vi "Select_events.vi"(8 "error in (no error)":errorcluster, 9 "Select errored events":bool, 10 "Small?":bool, 11 "Constraints":T1 {"Estimate Quality" scale=0.0..5.0; "Lower Mass Limit (kg)" min=-1.0 max=1.0 step=1e-20; "Upper Mass Limit (kg)" min=-1.0 max=1.0 step=1e-20; "Lower Velocity Limit (km/s)" min=-1.0 max=299792000.0; "Upper Velocity Limit (km/s)" min=-1.0 max=299792000.0}) -> (0 "error out":errorcluster, 3 "Dust Events":i64[](array[numeric]))   [LabVIEW 2013]
doc: "Selects the id's of all dust events that match the given constraints."
uses:
  User Interface/Controls/Constraints.ctl
  <vilib>/addons/database/_DB Variant To Data/Database Variant To Data.xnode
panel:
  out "Select Events Syntax":string
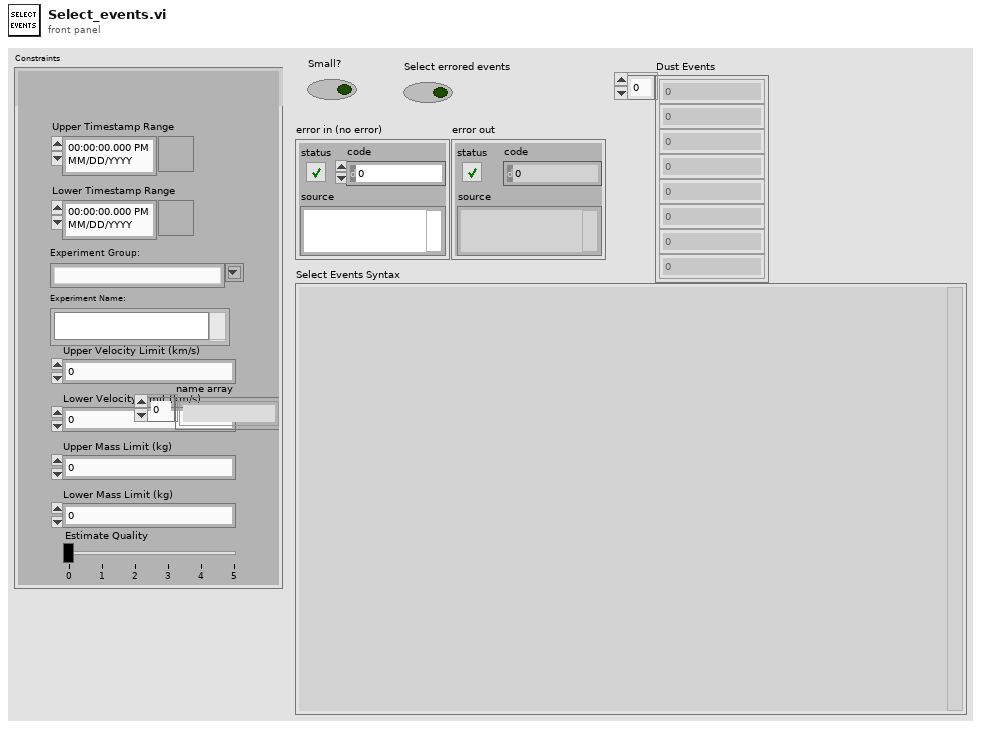
[diagram p1: front panel]
types:
  T1 = typedef "Constraints.ctl" = cluster{"Upper Timestamp Range":timestamp, "Lower Timestamp Range":timestamp, "Experiment Group:":string, "Experiment Name:":i32[], "Upper Velocity Limit (km/s)":dbl, "Lower Velocity Limit (km/s)":dbl, "Upper Mass Limit (kg)":dbl, "Lower Mass Limit (kg)":dbl, "name array":string[], "Estimate Quality":cluster{dbl, dbl}}
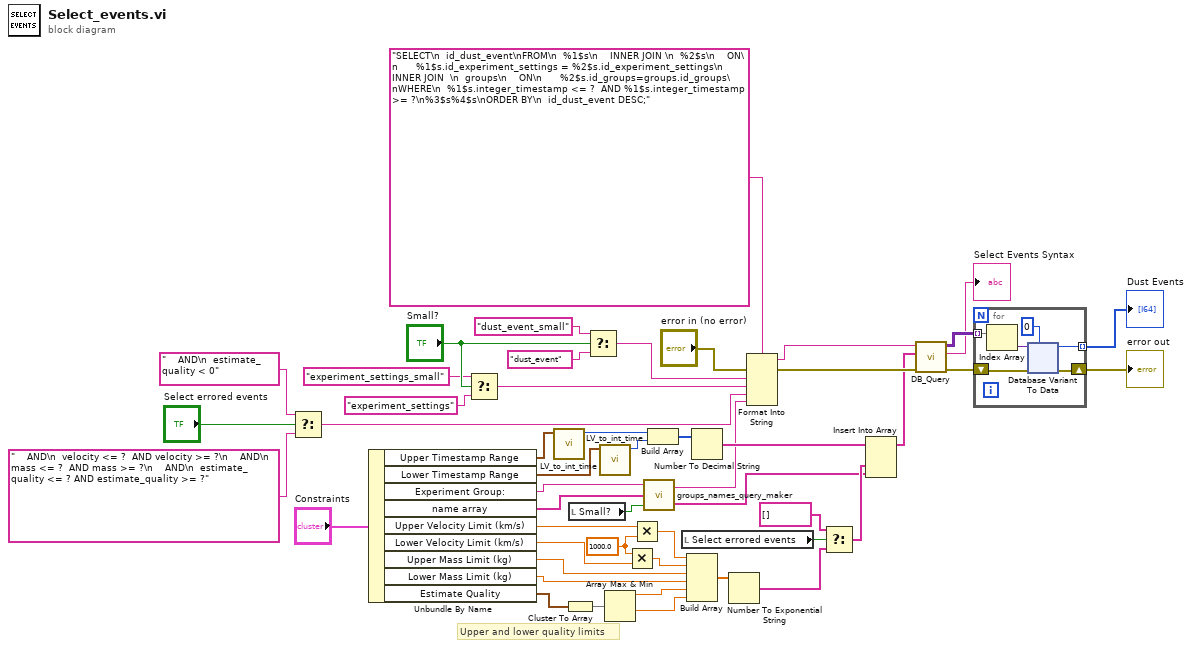
[diagram p0: block diagram]
diagram:
  w48 = 1000.0 ("y")
  # "Upper and lower quality limits"
  n1 = Select(t="    AND\n  estimate_quality < 0", s="Select errored events", f="    AND\n  velocity <= ?  AND velocity >= ?\n    AND\n  mass <= ?  AND mass >= ?\n    AND\n  estimate_quality <= ? AND estimate_quality >= ?" ("input 10")) -> (s? t:f=w3:string)
  n2 = Unbundle By Name("Constraints") -> ("Upper Timestamp Range"=w44:timestamp, "Lower Timestamp Range"=w43:timestamp, "Experiment Group:"=w30:string, "name array"=w29:string[], "Upper Velocity Limit (km/s)"=w39:dbl, "Lower Velocity Limit (km/s)"=w38:dbl, "Upper Mass Limit (kg)"=w34:dbl, "Lower Mass Limit (kg)"=w35:dbl, "Estimate Quality"=w46:cluster{dbl, dbl})
  n3 = Select(t="experiment_settings_small" ("Lower Mass Limit (kg)"), s="Small?", f="experiment_settings" ("Lower Mass Limit (kg)")) -> (s? t:f=w12:string)
  n4 = call "LV_to_int_time.vi"("Time Stamp"=w44) -> ("Integer Time"=w26:i64)  [unwired: 8 in, 1 out]
  n5 = Cluster To Array(cluster=w46) -> (array=w49:dbl[])
  n6 = local read "Small?"() -> (w28:bool)
  n7 = Select(t="dust_event_small" ("Lower Mass Limit (kg)"), s="Small?", f="dust_event" ("Lower Mass Limit (kg)")) -> (s? t:f=w11:string)
  n8 = call "LV_to_int_time.vi"("Time Stamp"=w43) -> ("Integer Time"=w25:i64)  [unwired: 8 in, 1 out]
  n9 = Array Max & Min(array=w49) -> (max value=w36:dbl, min value=w37:dbl)  [unwired: 2 out]
  n10 = Multiply(x=w48, y=w38) -> (x*y=w33:dbl)
  n11 = Multiply(x=w39, y=w48) -> (x*y=w32:dbl)
  n12 = call "groups_names_query_maker.vi"("Small?"=w28, "Name Array"=w29, "Group  Name"=w30) -> ("Parameters"=w1:string[], "Group and Names Query"=w4:string)
  n13 = Build Array(w26, w25) -> (w24:i64[])
  n14 = local read "Select errored events"() -> (w23:bool)
  n15 = Build Array(w32, w33, w34, w35, w36, w37) -> (w27:dbl[])
  n16 = Number To Decimal String(number=w24) -> (decimal integer string=w10:string[])  [unwired: 1 in]
  n17 = Number To Exponential String(number=w27) -> (E-format string=w20:string[])  [unwired: 3 in]
  n18 = Format Into String(format string="SELECT\n  id_dust_event\nFROM\n  %1$s\n    INNER JOIN \n  %2$s\n    ON\n      %1$s.id_experiment_settings = %2$s.id_experiment_settings\n    INNER JOIN  \n  groups\n    ON\n      %2$s.id_groups=groups.id_groups\nWHERE\n  %1$s.integer_timestamp <= ?  AND %1$s.integer_timestamp >= ?\n%3$s%4$s\nORDER BY\n  id_dust_event DESC;" ("string"), error in="error in (no error)", w11, w12, w3, w4) -> (resulting string=w8:string, error out=w18:errorcluster)  [unwired: 1 in]
  n19 = Select(t=string[] [] ("f"), s=w23, f=w20) -> (s? t:f=w2:string[])
  n20 = Insert Into Array(array=w10, new element #1=w2, new element #2=w1) -> (w9:string[])  [unwired: 1 in]
  n21 = call "DB_Query.vi"("error in (no error)"=w18, "Parameters"=w9, "Parameterized Query"=w8) -> ("error out"=w7:errorcluster, "Query in Standard Format"=→"Select Events Syntax":string, "Results"=w6:variant[][])  [unwired: 6 in]
  n22 = for {
    tunnel: [w53] -> w42 mode=indexing
    shift-right: [w54] -> w45
    shift-left: w7 -> [w55]
    tunnel: w6 -> [w50] mode=indexing
    n23 = Index Array(array=w50) -> (element=w52:variant)  [unwired: 1 in]
    n24 = xnode "Database Variant To Data"("database variant"=w52, "error in (no error)"=w55, "type"=i64 0 ("Number of Events")) -> ("data"=w53:i64, "error out"=w54:errorcluster)
  }
  "error out" <- w45
  "Dust Events" <- w42
